vi "RSZVB Read Trace Data.vi"(7 "Wait for OPC":bool, 8 "error in (no error)":errorcluster {"code" format="%.0x"}, 9 "Force ASCII":bool, 10 "Buffer":string, 11 "VISA session":refnum<visa-resource-name>) -> (0 "error out":errorcluster {"code" format="%.0x"}, 1 "Trace Data":dbl[](array[numeric]) format="%^.3e", 3 "dup VISA session":refnum<visa-resource-name>)   [LabVIEW 2015]
doc: "This VI reads out trace data from the instrument. It serves as utility VI.\n\nRemote-control command(s):\nFORMat[:DATA] ASCii | REAL64,"
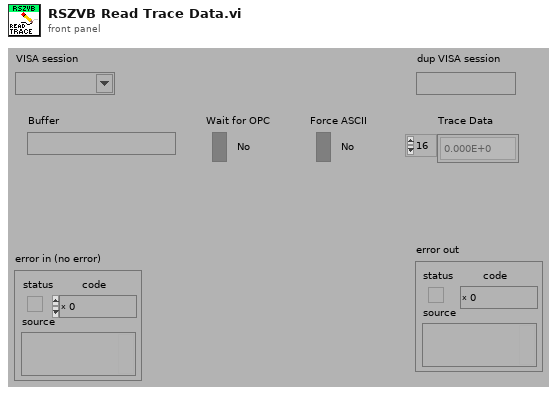
[diagram p1: front panel]
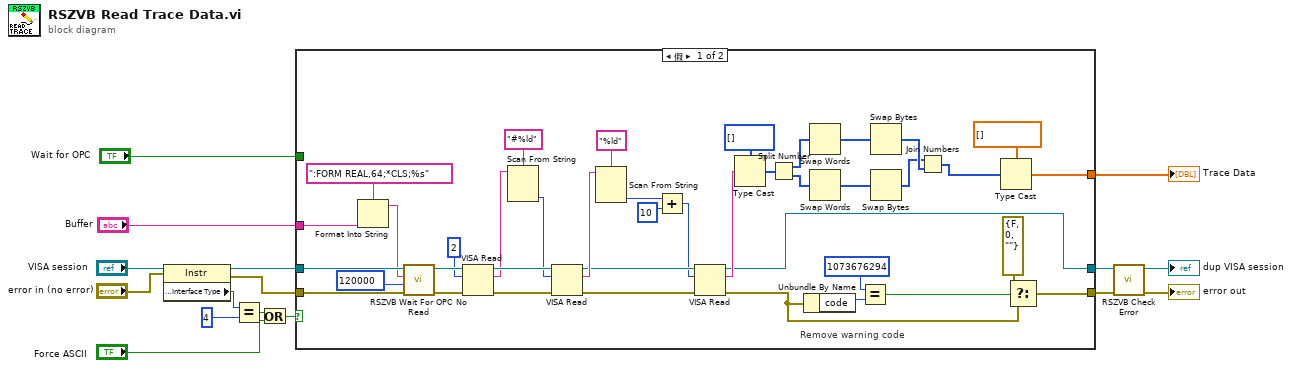
[diagram p0: block diagram]
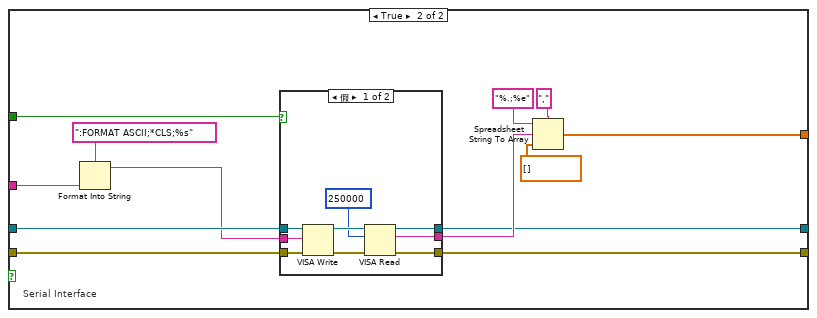
[diagram p2: hidden frame]
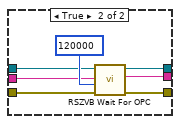
[diagram p3: hidden frame]
diagram:
  n1 = property class="Instr"(reference="VISA session", error in="error in (no error)") -> (reference out=w15:refnum<visa-resource-name>, error out=w16:errorcluster, "Interface Information:Interface Type"=w13:u16)
  n2 = Equal?(x=w13, y=u16 4) -> (x = y?=w4:bool)
  n3 = Or(x=w4, y="Force ASCII") -> (x .or. y?=w5:bool)
  n4 = case shown="假" w5 {
    tunnel: [w26 w59] -> w1
    tunnel: [w31 w60] -> w9
    tunnel: [w34 w61] -> w10
    tunnel: w15 -> [w54 w65]
    tunnel: w16 -> [w53 w64]
    tunnel: "Buffer" -> [w55 w58]
    tunnel: "Wait for OPC" -> [_ w57]
    frame False {
      # "Remove warning code"
      n5 = Format Into String(format string=":FORM REAL,64;*CLS;%s", w55) -> (resulting string=w52:string)  [unwired: 2 in, 1 out]
      n6 = call "RSZVB Wait For OPC No Read.vi"("error in (no error)"=w53, "Timeout (300000 ms)"=u32 120000, "Command"=w52, "VISA session"=w54) -> ("error out"=w51:errorcluster, "dup VISA session"=w50:refnum<visa-resource-name>)  [unwired: 6 in]
      n7 = VISA Read(VISA resource name=w50, byte count=u32 2, error in (no error)=w51) -> (VISA resource name out=w48:refnum<visa-resource-name>, read buffer=w45:string, error out=w47:errorcluster)  [unwired: 1 out]
      n8 = Scan From String(format string="#%ld", input string=w45) -> (output 1=w44:i32)  [unwired: 3 in, 3 out]
      n9 = VISA Read(VISA resource name=w48, byte count=w44, error in (no error)=w47) -> (VISA resource name out=w41:refnum<visa-resource-name>, read buffer=w42:string, error out=w40:errorcluster)  [unwired: 1 out]
      n10 = Scan From String(format string="%ld", input string=w42) -> (output 1=w25:i32)  [unwired: 3 in, 3 out]
      n11 = Add(x=w25, y=10) -> (x+y=w38:i32)
      n12 = VISA Read(VISA resource name=w41, byte count=w38, error in (no error)=w40) -> (VISA resource name out=w34:refnum<visa-resource-name>, read buffer=w36:string, error out=w29:errorcluster)  [unwired: 1 out]
      n13 = Type Cast(type=u64[] [], x=w36) -> (*(type *) &x=w23:u64[])
      n14 = Split Number(x=w23) -> (hi(x)=w21:u32[], lo(x)=w20:u32[])
      n15 = Unbundle By Name(w29) -> ("code"=w32:i32)
      n16 = Swap Words(1:w21) -> (0:w24:u32[])
      n17 = Swap Words(1:w20) -> (0:w22:u32[])
      n18 = Equal?(x=1073676294, y=w32) -> (x = y?=w30:bool)
      n19 = Swap Bytes(anything=w24) -> (byte swapped=w19:u32[])
      n20 = Swap Bytes(anything=w22) -> (byte swapped=w18:u32[])
      n21 = Join Numbers(hi=w18, lo=w19) -> ((hi.lo)=w17:u64[])
      n22 = Type Cast(type=dbl[] [], x=w17) -> (*(type *) &x=w26:dbl[])
      n23 = Select(t=errorcluster {"status"=FALSE, "code"=0, "source"=""} ("s? t:f"), s=w30, f=w29) -> (s? t:f=w31:errorcluster)
    }
    frame True {
      # "Serial Interface"
      n24 = Format Into String(format string=":FORMAT ASCII;*CLS;%s", w58) -> (resulting string=w62:string)  [unwired: 2 in, 1 out]
      n25 = case shown="假" w57 {
        tunnel: [w76 w80] -> w66
        tunnel: w65 -> [w75 w84]
        tunnel: w64 -> [w74 w83]
        tunnel: w62 -> [w73 w79]
        tunnel: [w72 w82] -> w61
        tunnel: [w71 w81] -> w60
        frame False {
          n26 = VISA Write(VISA resource name=w75, write buffer=w73, error in (no error)=w74) -> (VISA resource name out=w77:refnum<visa-resource-name>, error out=w78:errorcluster)  [unwired: 1 out]
          n27 = VISA Read(VISA resource name=w77, byte count=u32 250000 ("byte count (0)"), error in (no error)=w78) -> (VISA resource name out=w72:refnum<visa-resource-name>, read buffer=w76:string, error out=w71:errorcluster)  [unwired: 1 out]
        }
        frame True {
          n28 = call "RSZVB Wait For OPC.vi"("error in (no error)"=w83, "Timeout (300000 ms)"=u32 120000, "Command"=w79, "VISA session"=w84) -> ("error out"=w81:errorcluster, "Read Buffer"=w80:string, "dup VISA session"=w82:refnum<visa-resource-name>)  [unwired: 5 in]
        }
      }
      n29 = Spreadsheet String To Array(delimiter (Tab)=",", format string="%.;%e" ("delimiter (Tab)"), spreadsheet string=w66, array type (2D Dbl)=dbl[] [] ("Real Parts (I)")) -> (array=w59:dbl[])
    }
  }
  "Trace Data" <- w1
  n30 = call "RSZVB Check Error.vi"("error in (no error)"=w9, "VISA session"=w10) -> ("error out"=→"error out":errorcluster, "dup VISA session"=→"dup VISA session":refnum<visa-resource-name>)  [unwired: 8 in]
